vi "PreUUT.vi"(7 "Execution Data":variant, 8 "error in (no error)":errorcluster, 10 "Execution in":refnum<data-value>, 11 "TestProjectBase in":refnum<class "Project.lvclass">) -> (0 "error out":errorcluster, 2 "Execution out":refnum<data-value>, 3 "TestProjectBase out":refnum<class "Project.lvclass">)   [LabVIEW 2015, in "Project.lvclass"]
uses:
  Project.lvclass
  Execution.lvclass
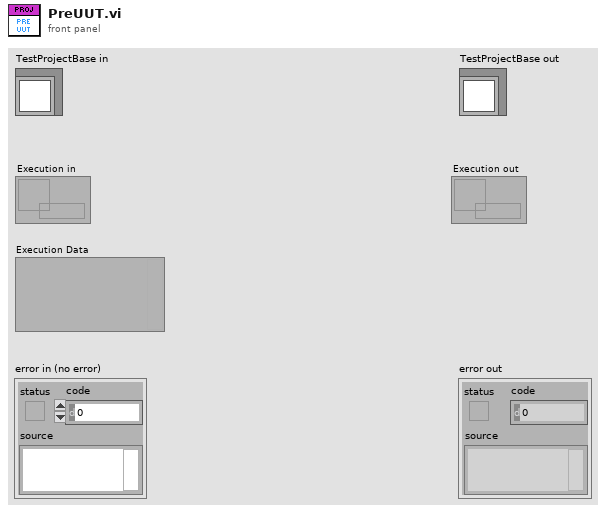
[diagram p1: front panel]
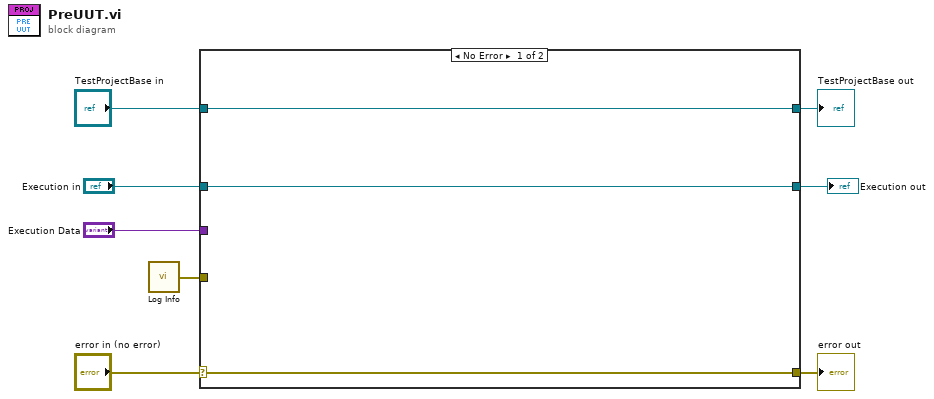
[diagram p0: block diagram]
diagram:
  n1 = call "Log Info.vi"() -> ("error out"=w4:errorcluster)  [unwired: 5 in]
  n2 = case shown="No Error" "error in (no error)" {
    selector: "error in (no error)" -> [w10 w14]
    tunnel: [w10 w14] -> w7
    tunnel: [w11 w13] -> w5
    tunnel: "TestProjectBase in" -> [w11 w13]
    tunnel: w4 -> [_ _]
    tunnel: "Execution in" -> [w9 w12]
    tunnel: [w9 w12] -> w2
    tunnel: "Execution Data" -> [_ _]
    frame No Error {
    }
    frame Error {
    }
  }
  "error out" <- w7
  "TestProjectBase out" <- w5
  "Execution out" <- w2
